vi "Unset Method Library Tag.vi"(8 "error in (no error)":errorcluster, 9 "Message Type":T1, 11 "LVClassLibrary in":refnum<vi>) -> (0 "error out":errorcluster, 3 "LVClassLibrary out":refnum<vi>)   [LabVIEW 2023, in "Message Maker.lvclass"]
uses:
  Message Type.ctl
  Message Maker.lvclass
  Message Maker.lvclass/Message Maker.ctl
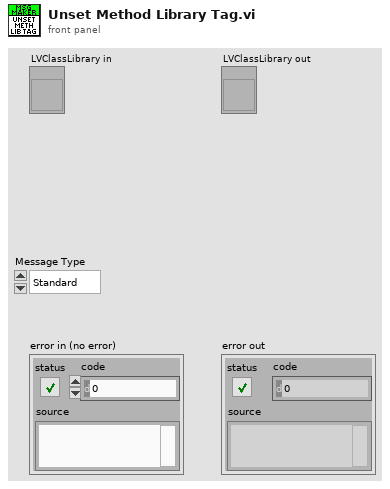
[diagram p1: front panel]
types:
  T1 = typedef "Message Maker.lvclass/Message Type.ctl" = enum16{"Standard", "Async"}
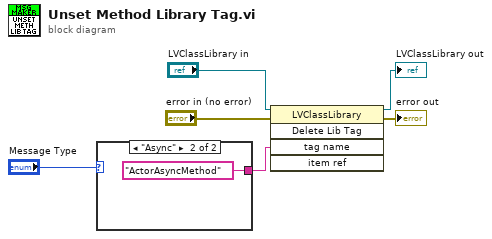
[diagram p0: block diagram]
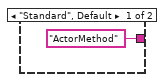
[diagram p2: hidden frame]
diagram:
  n1 = case shown="\"Async\"" "Message Type" {
    tunnel: ["ActorMethod" ("Tag Name") "ActorAsyncMethod" ("Tag Name")] -> w6
    frame "Standard", Default {
    }
    frame "Async" {
    }
  }
  n2 = invoke class="LVClassLibrary" method="Delete Lib Tag"(reference="LVClassLibrary in", error in="error in (no error)", "tag name"=w6) -> (reference out=→"LVClassLibrary out":refnum<vi>, error out=→"error out":errorcluster)  [unwired: 2 in, 3 out]
